vi "remove_zero_rows.vi"(1 "all rows in":dbl[][](array[numeric])) -> (0 "all rows out":dbl[][](array[numeric]))   [LabVIEW 2012]
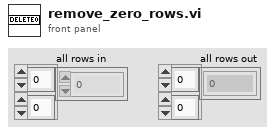
[diagram p1: front panel]
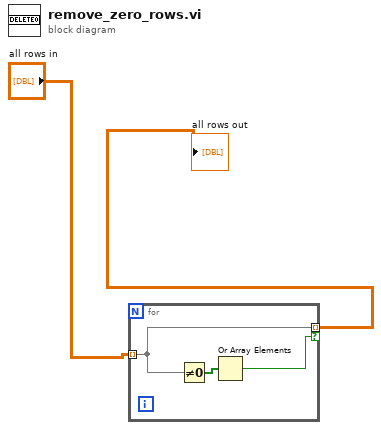
[diagram p0: block diagram]
diagram:
  n1 = for {
    tunnel: "all rows in" -> [w5] mode=indexing
    tunnel: [w5] -> w2 mode=indexing if=w4
    n2 = Not Equal To 0?(x=w5) -> (x != 0?=w3:bool[])
    n3 = Or Array Elements(Boolean array=w3) -> (logical OR=w4:bool)
  }
  "all rows out" <- w2
